vi "Prober_CloseSession.vi"(8 "error in (no error)":errorcluster, 11 "SemiProbe in":refnum<class "SemiProbe.lvclass">) -> (0 "error out":errorcluster, 3 "SemiProbe out":refnum<class "SemiProbe.lvclass">)   [LabVIEW 2019, in "SemiProbe.lvclass"]
uses:
  SemiProbe.lvclass
  Protected/SP_BusyCheck.vi
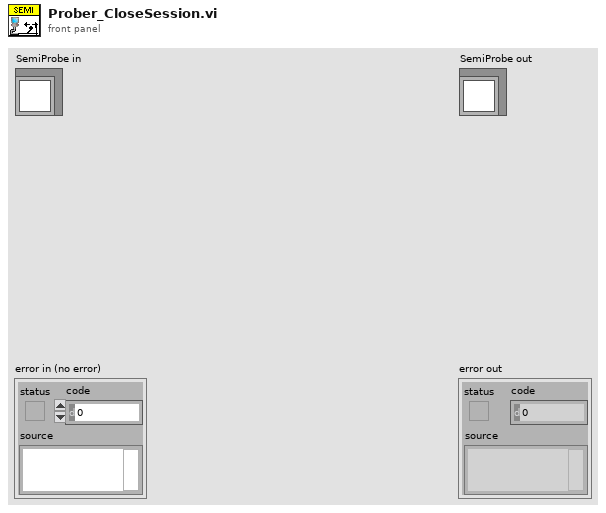
[diagram p1: front panel]
types:
  T1 = cluster{"SemiProbe VISA":refnum<visa-resource-name>, "write delay(ms)":i32, "buffer is full loop multiplicity":i32, "read threshold check rate (ms)":u32}
  T2 = cluster{"address":string, "port":i32, "SP TCP Cnx ID":refnum<k5>, "mode (standard)":enum16{"Standard", "Buffered", "CRLF", "Immediate"}, "bytes to read":i32, "timeout (ms)":i32}
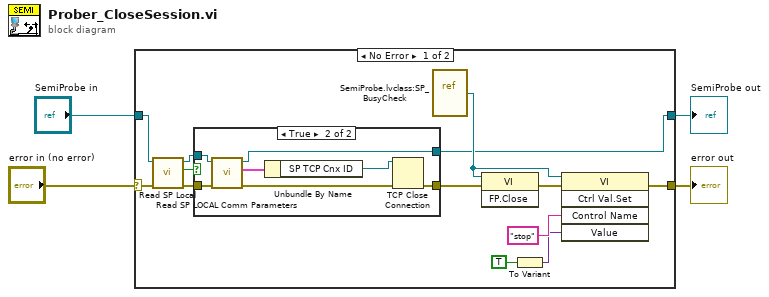
[diagram p0: block diagram]
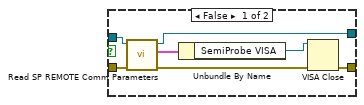
[diagram p2: hidden frame]
diagram:
  n1 = case shown="No Error" "error in (no error)" {
    selector: "error in (no error)" -> [w12 w33]
    tunnel: [w6 w33] -> w3
    tunnel: "SemiProbe in" -> [w13 w32]
    tunnel: [w5 w32] -> w1
    frame No Error {
      n2 = call-dynamic "Read SP Local.vi"("error in (no error)"=w12, "SemiProbe in"=w13) -> ("error out"=w10:errorcluster, "SP Local"=w11:bool, "SemiProbe out"=w9:refnum<class "SemiProbe.lvclass">)  [unwired: 7 in]
      n3 = case shown="True" w11 {
        tunnel: w10 -> [w23 w31]
        tunnel: w9 -> [w24 w30]
        tunnel: [w19 w25] -> w8
        tunnel: [w18 w27] -> w5
        frame False {
          n4 = call-dynamic "Read SP REMOTE Comm Parameters.vi"("error in (no error)"=w23, "SemiProbe in"=w24) -> ("error out"=w20:errorcluster, "SP REMOTE Comm Parameters"=w22:T1, "SemiProbe out"=w18:refnum<class "SemiProbe.lvclass">)  [unwired: 7 in]
          n5 = Unbundle By Name(w22) -> ("SemiProbe VISA"=w21:refnum<visa-resource-name>)
          n6 = VISA Close(VISA resource name=w21, error in (no error)=w20) -> (error out=w19:errorcluster)
        }
        frame True {
          n7 = call-dynamic "Read SP LOCAL Comm Parameters.vi"("error in (no error)"=w31, "SemiProbe in"=w30) -> ("error out"=w28:errorcluster, "SP LOCAL Comm Parameters"=w29:T2, "SemiProbe out"=w27:refnum<class "SemiProbe.lvclass">)  [unwired: 7 in]
          n8 = Unbundle By Name(w29) -> ("SP TCP Cnx ID"=w26:refnum<k5>)
          n9 = TCP Close Connection(connection ID=w26, error in (no error)=w28) -> (error out=w25:errorcluster)  [unwired: 1 in, 1 out]
        }
      }
      n10 = vi-ref "SemiProbe.lvclass:SP_BusyCheck.vi"() -> (w17:refnum<vi>)
      n11 = invoke class="VI" method="FP.Close"(reference=w17, error in=w8) -> (error out=w7:errorcluster)  [unwired: 1 in, 2 out]
      n12 = To Variant(anything=TRUE) -> (Variant=w14:variant)
      n13 = invoke class="VI" method="Ctrl Val.Set"(reference=w17, error in=w7, "Control Name"="stop", "Value"=w14) -> (error out=w6:errorcluster)  [unwired: 1 in, 4 out]
    }
    frame Error {
    }
  }
  "error out" <- w3
  "SemiProbe out" <- w1
